vi "MOKE-5-3-22.vi"() -> ()   [LabVIEW 2020]
uses:
  <vilib>/Analysis/Matrix/Datatypes/RealMatrix.ctl
  <vilib>/Analysis/baseanly.llb/Mean (DBL).vi
  <vilib>/Analysis/NI_AALBase.lvlib
  <vilib>/Analysis/Matrix/NI_Matrix.lvlib
panel:
  out "photodiode live avg graph (plots every average, need to update)":cluster{"Y":dbl[], "Y":dbl[]}[](graph)
  out "photodiode final avg graph":cluster{"Y":dbl[], "Y":dbl[]}[](graph)
  out "avgs  (missing last two values but that's ok ig)":dbl[](array[numeric])
  out "avg":dbl
  out "col_arr":dbl[][](array[numeric])
  in  "blank":dbl[](array[numeric])
  out "y_mat":T1
  in  "stop":bool
  in  "Total Loops":dbl
  out "Current Loop":i32
  in  "Time / Step":i64
  in  "Number of Samples":i32=100
  out "Graph For Photodiode":cluster{"Y":dbl[], "Y":dbl[]}[](graph)
  out "Photodiode Level":dbl
  out "Current Voltage":dbl
  in  "Scans From 0 to Max Voltage":i32
  in  "Voltage":dbl
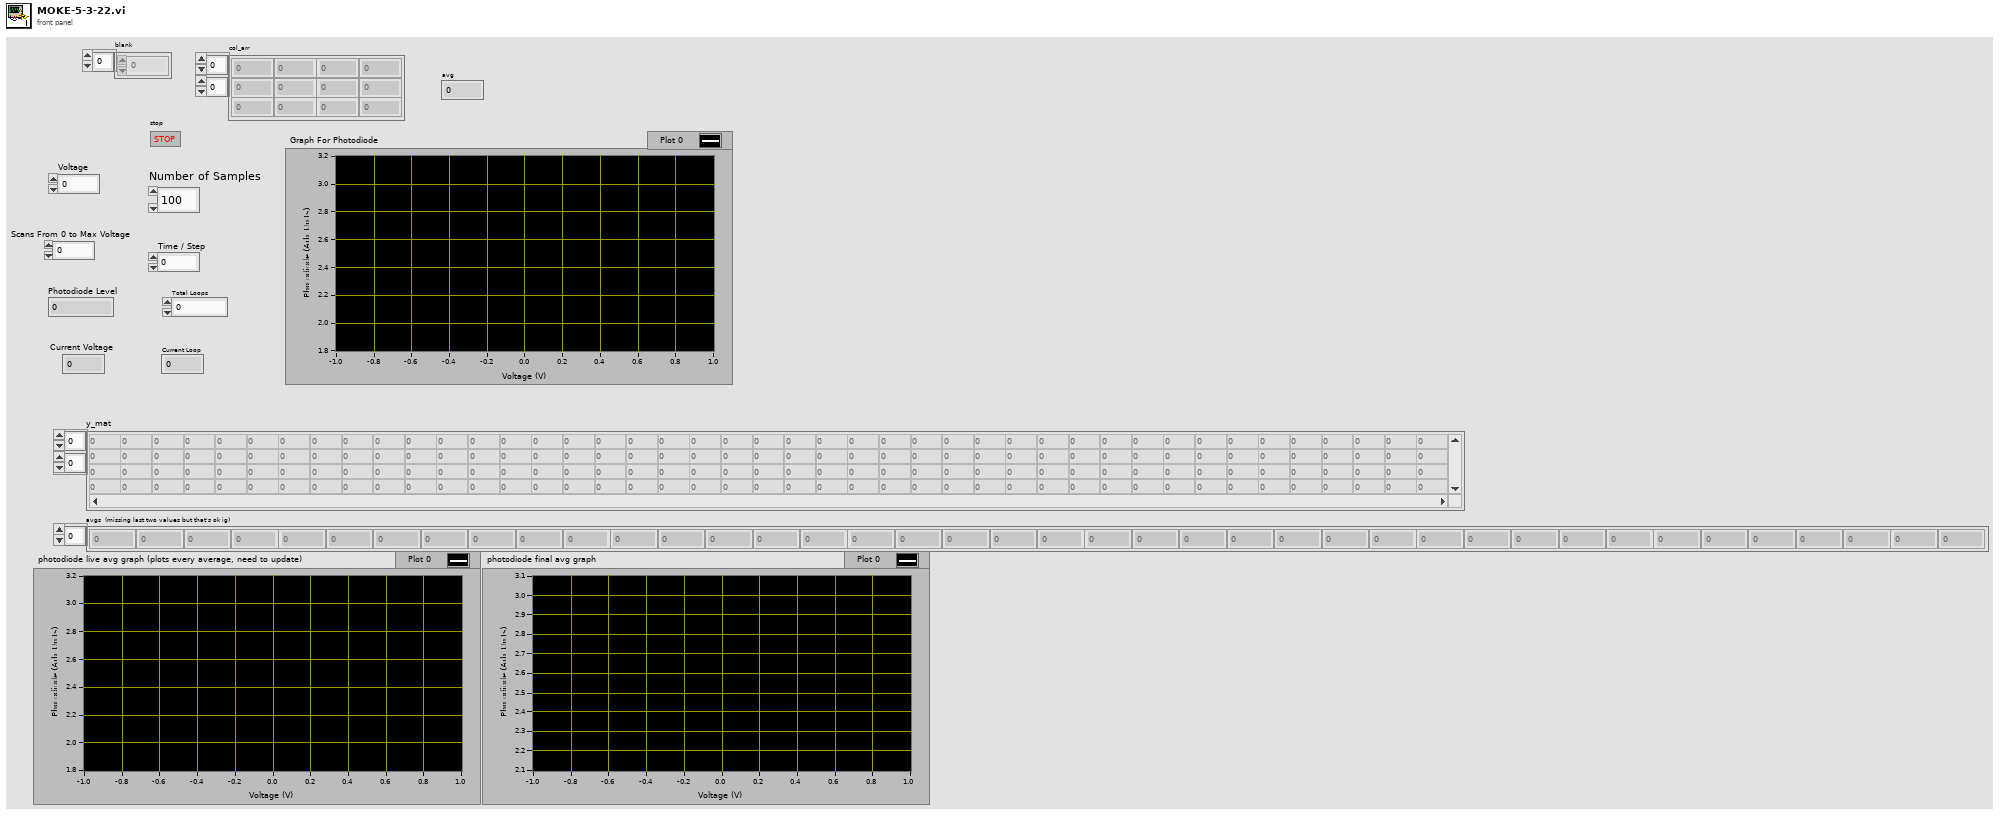
[diagram p1: front panel]
types:
  T1 = typedef "NI_Matrix.lvlib/RealMatrix.ctl" = dbl[][]
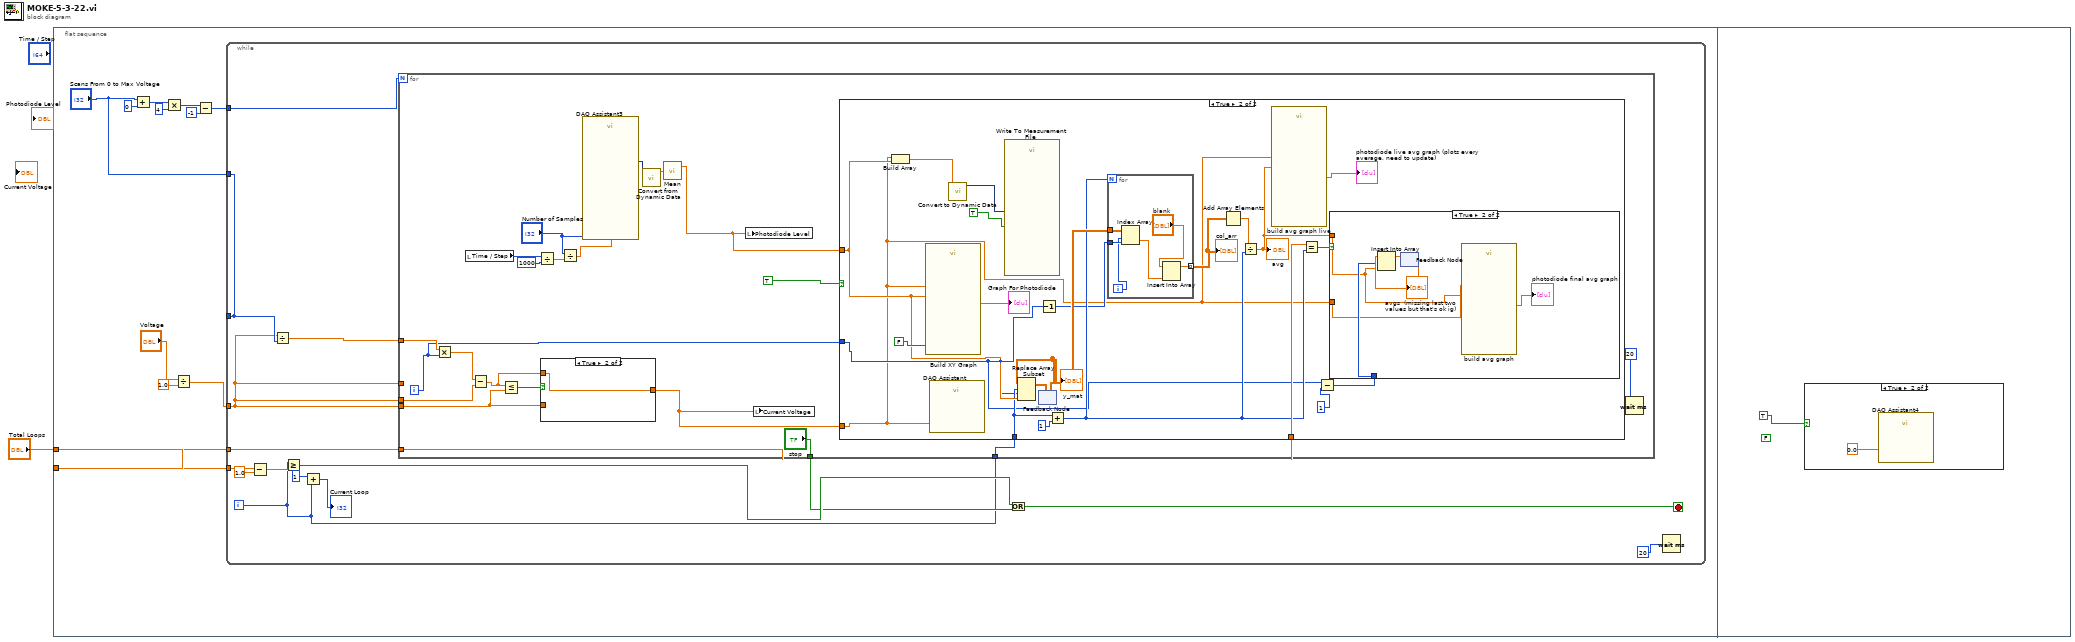
[diagram p0: block diagram]
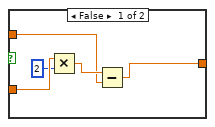
[diagram p2: hidden frame]
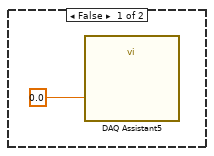
[diagram p5: hidden frame]
diagram:
  n1 = flat-sequence {
    tunnel: "Total Loops" -> [w6]
    tunnel: "Total Loops" -> [w2]
    frame #0 {
      n2 = Add(x="Scans From 0 to Max Voltage", y=0) -> (x+y=w12:i32)
      n3 = Multiply(x=w12, y=4) -> (x*y=w13:i32)
      n4 = Divide(x="Voltage", y=1.0) -> (x/y=w3:dbl)
      n5 = Subtract(x=w13, y=-1) -> (x-y=w8:i32)
      n6 = while {
        tunnel: w6 -> [w27]
        tunnel: [w18] -> _
        tunnel: w8 -> [w19]
        tunnel: "Scans From 0 to Max Voltage" -> [w18]
        tunnel: w3 -> [w17]
        tunnel: w2 -> [w14]
        i -> [w15]
        stop <- w21 stop-if-true
        n7 = Subtract(x=w27, y=1.0) -> (x-y=w26:dbl)
        n8 = Divide(x=w17, y=w18) -> (x/y=w28:dbl)
        n9 = Greater Or Equal?(x=w15, y=w26) -> (x >= y?=w22:bool)
        n10 = Add(x=1, y=w15) -> (x+y=→"Current Loop":i32)
        n11 = for {
          N: w19 -> [_]
          tunnel: w28 -> [w49]
          tunnel: w17 -> [_]
          tunnel: w17 -> [w46]
          tunnel: w17 -> [w42]
          tunnel: ["stop"] -> w20
          tunnel: w15 -> [w30]
          tunnel: w14 -> [w29]
          i -> [w31]
          n12 = Multiply(x=w49, y=w31) -> (x*y=w47:dbl)
          n13 = local read "Time / Step"() -> (w38:i64)
          n14 = Subtract(x=w47, y=w46) -> (x-y=w44:dbl)
          n15 = Less Or Equal?(x=w44, y=w42) -> (x <= y?=w45:bool)
          n16 = Divide(x=w38, y=i64 1000) -> (x/y=w39:dbl)
          n17 = case shown="True" w45 {
            tunnel: w44 -> [w51 w55]
            tunnel: [w50 w55] -> w43
            tunnel: w42 -> [w54 _]
            frame False {
              n18 = Multiply(x=w54, y=2) -> (x*y=w52:dbl)
              n19 = Subtract(x=w52, y=w51) -> (x-y=w50:dbl)
            }
            frame True {
            }
          }
          n20 = Divide(x="Number of Samples", y=w39) -> (x/y=w40:dbl)
          n21 = call "DAQ Assistant3"("rate"=w40, "number of samples"="Number of Samples") -> ("data"=w36:dynamicdata)  [unwired: 4 in, 13 out]
          n22 = call "Convert from Dynamic Data"("Dynamic Data Type"=w36) -> ("Array"=w35:dbl[])  [unwired: 3 in]
          n23 = call-poly <vilib>:"Mean.vi"("X"=w35) -> ("mean"=w34:dbl)  [unwired: 1 out]
          n24 = local write "Photodiode Level"(w34) -> ()
          n25 = local write "Current Voltage"(w43) -> ()
          n26 = case shown="True" TRUE {
            tunnel: w43 -> [_ w58]
            tunnel: w34 -> [_ w72]
            tunnel: w31 -> [_ w59]
            tunnel: w30 -> [_ w66]
            tunnel: w29 -> [_ w65]
            frame False {
            }
            frame True {
              n27 = Build Array(w58, w72) -> (w75:dbl[])
              n28 = call "Build XY Graph"("Reset"=FALSE, "Y Input"=w72, "X Input"=w58) -> ("XY Graph"=→"Graph For Photodiode":cluster{"X":dbl[], "Y":dbl[]}[])  [unwired: 7 in, 1 out]
              n29 = call "DAQ Assistant"("data"=w58) -> ()  [unwired: 17 in, 2 out]
              n30 = call "Convert to Dynamic Data"("Array"=w75) -> ("Dynamic Data Type"=w73:dynamicdata)  [unwired: 3 in]
              n31 = call "Write To Measurement File"("Signals"=w73, "Enable"=TRUE) -> ()  [unwired: 15 in, 3 out]
              n32 = feedback #1() -> (w70:T1)  [unwired: 1 in]
              "y_mat" <- w70
              n33 = Replace Array Subset(array=w70, new element=w72, index (row)=w66, index (col)=w59) -> (w71:T1)
              n34 = feedback-in #1(w71) -> ()
              n35 = Decrement(x=w59) -> (x-1=w60:i32)
              n36 = Add(x=w66, y=1) -> (x+y=w61:i32)
              n37 = for {
                N: w61 -> [_]
                tunnel: w70 -> [w89]
                tunnel: w60 -> [w85]
                tunnel: [w86] -> w69 mode=indexing
                i -> [w84]
                n38 = Index Array(array=w89, index (row)=w84, index (col)=w85) -> (element=w88:dbl)
                n39 = Insert Into Array(array="blank", new element=w88) -> (w86:dbl[])  [unwired: 1 in]
              }
              "col_arr" <- w69
              n40 = Add Array Elements(numeric array=w69) -> (sum=w68:dbl)
              n41 = Divide(x=w68, y=w61) -> (x/y=w57:dbl)
              "avg" <- w57
              n42 = call "build avg graph live"("Y Input"=w57, "X Input"=w58) -> ("XY Graph"=→"photodiode live avg graph (plots every average, need to update)":cluster{"X":dbl[], "Y":dbl[]}[])  [unwired: 8 in, 1 out]
              n43 = Equal?(x=w65, y=w61) -> (x = y?=w64:bool)
              n44 = Subtract(x=w59, y=1) -> (x-y=w63:i32)
              n45 = case shown="True" w64 {
                tunnel: w57 -> [_ w79]
                tunnel: w63 -> [_ w81]
                tunnel: w58 -> [_ w80]
                frame False {
                }
                frame True {
                  n46 = feedback #2() -> (w82:dbl[])  [unwired: 1 in]
                  "avgs  (missing last two values but that's ok ig)" <- w82
                  n47 = Insert Into Array(array=w82, index=w81, new element=w79) -> (w83:dbl[])
                  n48 = feedback-in #2(w83) -> ()
                  n49 = call "build avg graph"("Y Input"=w79, "X Input"=w80) -> ("XY Graph"=→"photodiode final avg graph":cluster{"X":dbl[], "Y":dbl[]}[])  [unwired: 8 in, 1 out]
                }
              }
            }
          }
          n50 = Wait (ms)(milliseconds to wait=20) -> ()  [unwired: 1 out]
        }
        n51 = Or(x=w22, y=w20) -> (x .or. y?=w21:bool)
        n52 = Wait (ms)(milliseconds to wait=u32 20) -> ()  [unwired: 1 out]
      }
    }
    frame #1 {
      (unwired) FALSE
      n53 = case shown="True" TRUE {
        frame False {
          n54 = call "DAQ Assistant5"("data"=0.0) -> ()  [unwired: 17 in, 2 out]
        }
        frame True {
          n55 = call "DAQ Assistant4"("data"=0.0) -> ()  [unwired: 17 in, 2 out]
        }
      }
    }
  }
